vi "To XML - Adds XML Entities.vi"() -> ()   [LabVIEW 2017, in "Cobertura.Tests.lvlib" / "Method.lvlib"]
uses:
  Method.lvlib
  <vilib>/xml/Close Reference(Node).vi
  Cobertura/Method/Method.lvclass
  <vilib>/xml/NI_XML.lvlib
  <resource>/objmgr/DOMUserDefRef.rc
  <vilib>/PNR/Transparent Assertions/Transparent Assertions/Transparent Assertions.lvlib
panel:
  out "error out":errorcluster
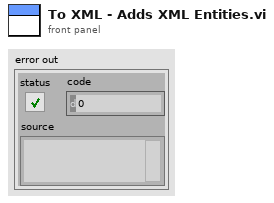
[diagram p1: front panel]
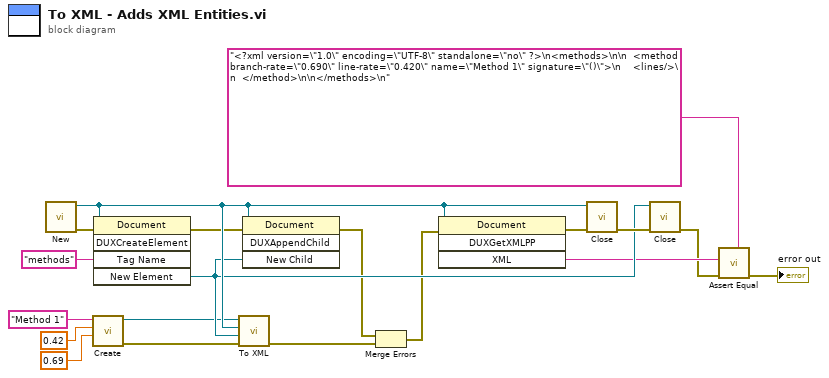
[diagram p0: block diagram]
diagram:
  n1 = call <vilib>:"New.vi"() -> ("error out"=w15:errorcluster, "DOM document out"=w17:refnum<k20>)  [unwired: 8 in]
  n2 = call "Create.vi"("Branch Rate"=0.69, "Line Rate"=0.42, "Name"="Method 1") -> ("error out"=w1:errorcluster, "Method"=w2:refnum<class "Method.lvclass">)  [unwired: 7 in]
  n3 = invoke class="Document" method="DUXCreateElement"(reference=w17, error in=w15, "Tag Name"="methods") -> (error out=w16:errorcluster, "New Element"=w13:refnum<k20>)  [unwired: 2 in, 3 out]
  n4 = call-dynamic "To XML.vi"("error in (no error)"=w1, "Parent"=w13, "Document"=w17, "Method in"=w2) -> ("error out"=w7:errorcluster)  [unwired: 7 in]
  n5 = invoke class="Document" method="DUXAppendChild"(reference=w17, error in=w16, "New Child"=w13) -> (error out=w9:errorcluster)  [unwired: 1 in, 3 out]
  n6 = Merge Errors(w9, w7) -> (w8:errorcluster)
  n7 = invoke class="Document" method="DUXGetXMLPP"(reference=w17, error in=w8) -> (error out=w18:errorcluster, "XML"=w12:string)  [unwired: 2 in, 2 out]
  n8 = call-poly <vilib>:"Close.vi"("error in (no error)"=w18, "node"=w17) -> ("error out"=w14:errorcluster)  [unwired: 7 in]
  n9 = call-poly <vilib>:"Close.vi"("error in (no error)"=w14, "node"=w13) -> ("error out"=w6:errorcluster)  [unwired: 7 in]
  n10 = call <vilib>:"Assert Equal.vi"("Expected"="<?xml version=\"1.0\" encoding=\"UTF-8\" standalone=\"no\" ?>\n<methods>\n\n  <method branch-rate=\"0.690\" line-rate=\"0.420\" name=\"Method 1\" signature=\"()\">\n    <lines/>\n  </method>\n\n</methods>\n", "error in (no error)"=w6, "Actual"=w12) -> ("error out"=→"error out":errorcluster)  [unwired: 8 in]
